vi "UpdateIndex.vi"() -> ()   [LabVIEW 2020]
panel:
  out "standard error":string
  out "String":string
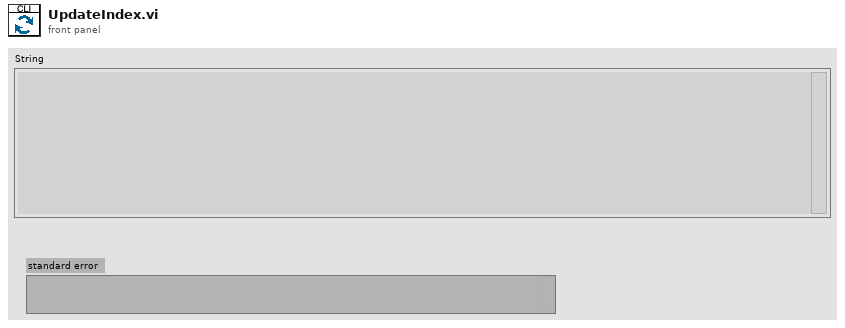
[diagram p1: front panel]
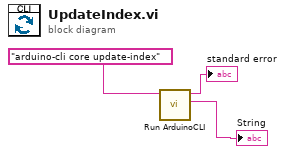
[diagram p0: block diagram]
diagram:
  n1 = call "Run ArduinoCLI.vi"("command line"="arduino-cli core update-index") -> ("standard output"=→"String":string, "standard error"=→"standard error":string)  [unwired: 9 in]
